vi "GFITS_Write3DHdrs.vi"(8 "error in (no error)":errorcluster, 10 "keys":string[][][](array[string]), 11 "fref":u64) -> (0 "error out":errorcluster)   [LabVIEW 2016]
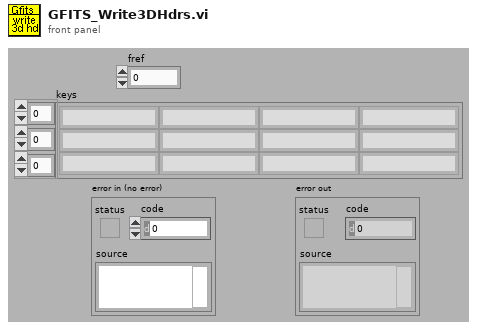
[diagram p1: front panel]
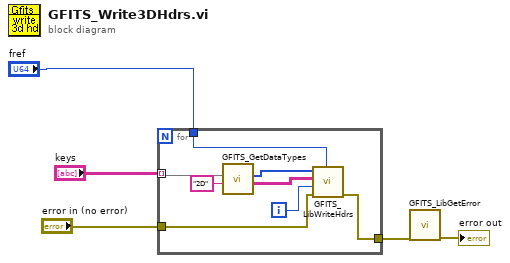
[diagram p0: block diagram]
diagram:
  n1 = for {
    tunnel: "keys" -> [w10] mode=indexing
    tunnel: "fref" -> [w9]
    tunnel: "error in (no error)" -> [w7]
    tunnel: [w6] -> w2
    i -> [w8]
    n2 = call "GFITS_GetDataTypes.vi"("type"="2D", "keys"=w10) -> ("keys out"=w12:string[][], "datatypes"=w11:i32[])  [unwired: 8 out]
    n3 = call "GFITS_LibWriteHdrs.vi"("file ref"=w9, "error in (no error)"=w7, "dnum"=w8, "Table In"=w12, "data type"=w11) -> ("error out"=w6:errorcluster)  [unwired: 6 out]
  }
  n4 = call "GFITS_LibGetError.vi"("error in (no error)"=w2) -> ("error out"=→"error out":errorcluster)  [unwired: 10 out]
